vi "阿基米德螺旋线.vi"() -> ()   [LabVIEW 2012]
uses:
  <vilib>/gmath/NI_Gmath.lvlib
panel:
  in  "Cycle(n*2pi)":dbl=5.0
  out "XY图":cluster{"X":dbl[], "Y":dbl[]}(graph)
  in  "radius as function of angle":string="2*t+1" caption="极径（极角的函数）"
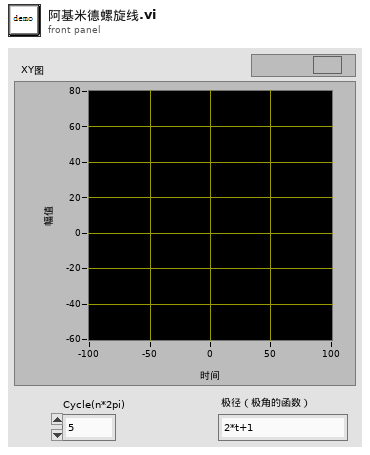
[diagram p1: front panel]
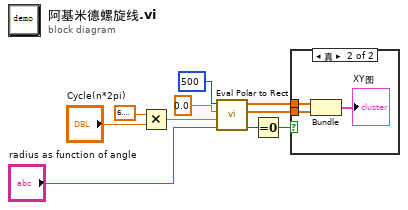
[diagram p0: block diagram]
diagram:
  n1 = Multiply(x=6.283185307179586, y="Cycle(n*2pi)") -> (x*y=w3:dbl)
  n2 = call <vilib>:"Eval Polar to Rect.vi"("radius as function of angle"="radius as function of angle", "end"=w3, "start"=0.0, "number of points"=u32 500) -> ("error"=w2:i32, "Y"=w8:dbl[], "X"=w9:dbl[])  [unwired: 1 out]
  n3 = Equal To 0?(x=w2) -> (x = 0?=w1:bool)
  n4 = case shown="真" w1 {
    tunnel: w9 -> [_ w13]
    tunnel: w8 -> [_ w12]
    frame False {
    }
    frame True {
      n5 = Bundle("X"=w13, "Y"=w12) -> (→"XY图":cluster{"X":dbl[], "Y":dbl[]})  [unwired: 1 in]
    }
  }
